vi "Graph test.vi"() -> ()   [LabVIEW 2024]
panel:
  out "XY Graph":cluster{"X":dbl, "Y":dbl}[](graph)
  out "Waveform Graph 2":cluster{dbl, dbl, dbl[]}(graph)
  out "Waveform Chart":cluster{dbl, dbl}(graph)
  out "Waveform Graph":dbl[](graph)
  in  "stop":bool
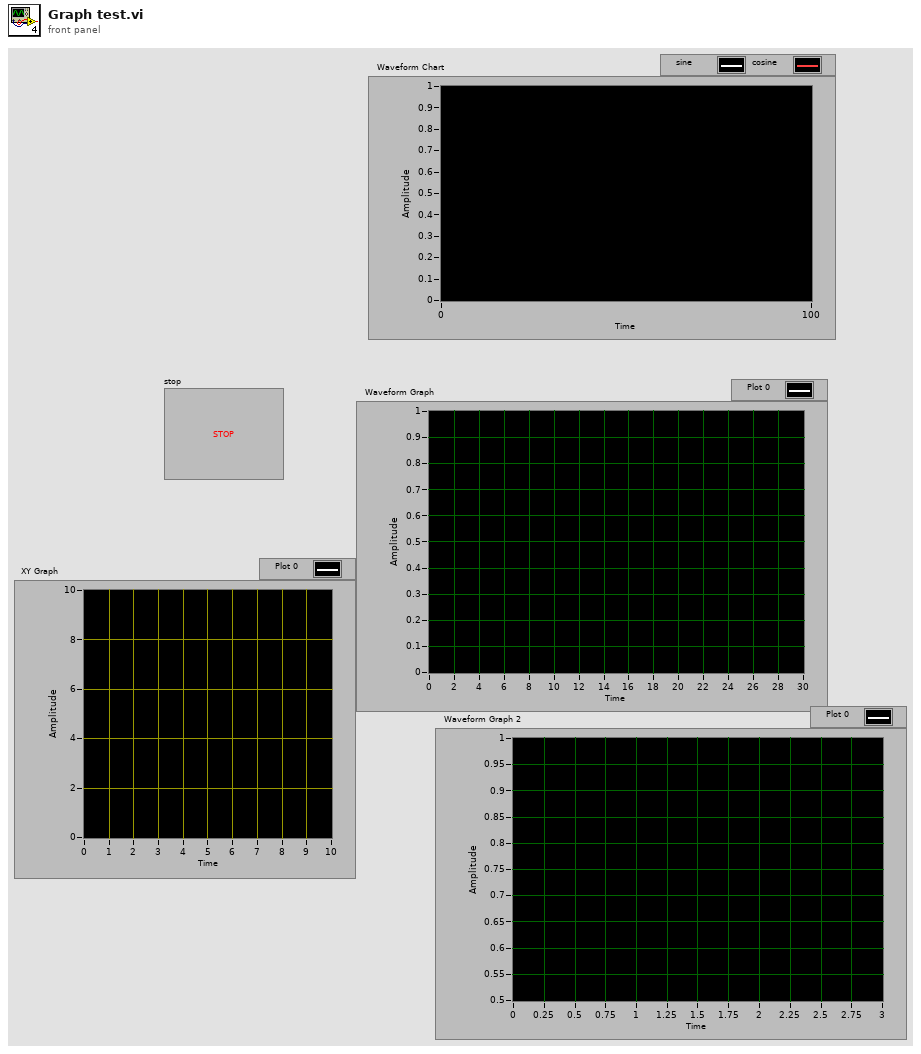
[diagram p1: front panel]
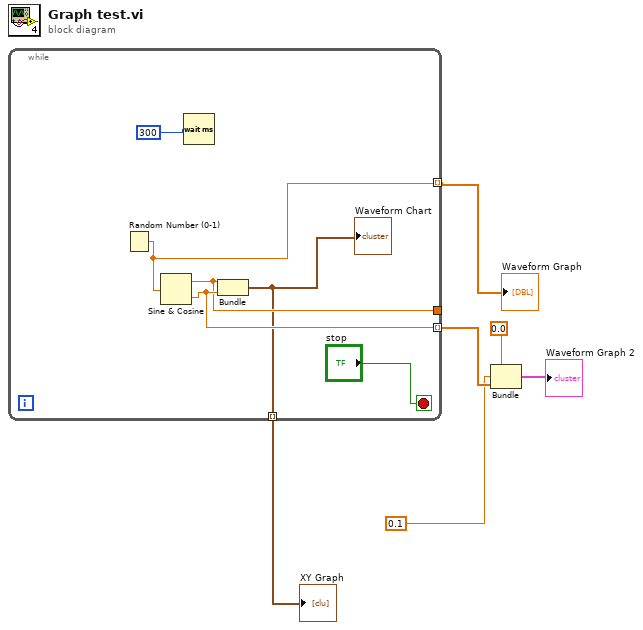
[diagram p0: block diagram]
diagram:
  n1 = while {
    tunnel: [w10] -> w3 mode=indexing
    tunnel: [w9] -> _
    tunnel: [w8] -> w6 mode=indexing
    tunnel: [w7] -> w1 mode=indexing
    stop <- "stop" stop-if-true
    n2 = Random Number (0-1)() -> (number: 0 to 1=w8:dbl)
    n3 = Sine & Cosine(0:w8) -> (1:w9:dbl, 2:w10:dbl)
    n4 = Wait (ms)(milliseconds to wait=u32 300) -> ()  [unwired: 1 out]
    n5 = Bundle(w9, w10) -> (w7:cluster{dbl, dbl})  [unwired: 1 in]
    "Waveform Chart" <- w7
  }
  "Waveform Graph" <- w6
  "XY Graph" <- w1
  n6 = Bundle(0.0, 0.1, w3) -> (→"Waveform Graph 2":cluster{dbl, dbl, dbl[]})  [unwired: 1 in]
